vi "ProcessTimestamp.vi"(10 "Action":T1, 11 "Original":string) -> (3 "Processed":string)   [LabVIEW 2020]
uses:
  TimestampAction.ctl
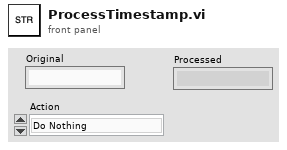
[diagram p1: front panel]
types:
  T1 = typedef "TimestampAction.ctl" = enum16{"Do Nothing", "Remove T"}
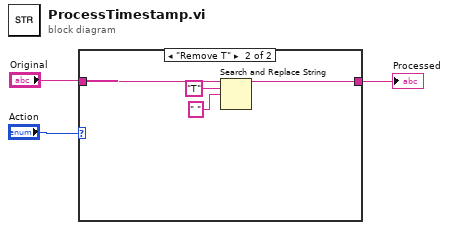
[diagram p0: block diagram]
diagram:
  n1 = case shown="\"Remove T\"" "Action" {
    tunnel: "Original" -> [w4 w6]
    tunnel: [w4 w5] -> w1
    frame "Do Nothing", Default {
    }
    frame "Remove T" {
      n2 = Search and Replace String(input string=w6, search string="T", replace string=" " ("replace string (\"\")")) -> (result string=w5:string)  [unwired: 5 in, 3 out]
    }
  }
  "Processed" <- w1
